vi "LWXPS_SetZone.vi"(5 "LabVIEW error IN":errorcluster, 6 "XPS Reference IN":refnum<k24>, 7 "Hysteresis":dbl, 8 "Radius":dbl, 9 "Y center":dbl, 10 "X center":dbl) -> (0 "LabVIEW error OUT":errorcluster, 1 "XPS Error String":string, 2 "Returned error code":i32, 3 "XPS Reference OUT":refnum<k24>)   [LabVIEW 2014]
uses:
  D:/XPSQ8_LabView_Library/Development/Source/Dll/Newport.XPS.CommandInterface.dll
  Dll/Newport.XPS.CommandInterface.dll
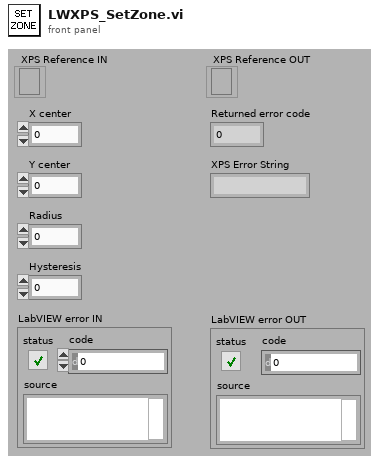
[diagram p1: front panel]
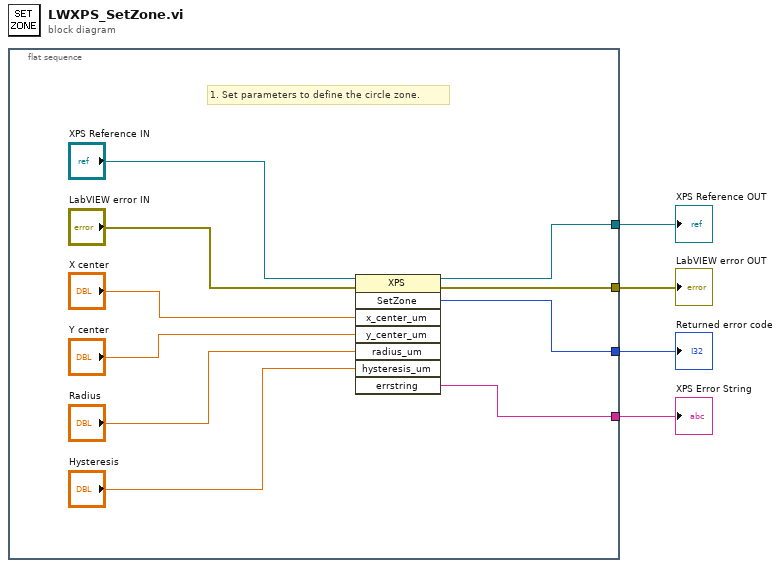
[diagram p0: block diagram]
diagram:
  n1 = flat-sequence {
    tunnel: [w11] -> w4
    tunnel: [w10] -> w3
    tunnel: [w12] -> w2
    tunnel: [w7] -> w1
    frame #0 {
      # "1. Set parameters to define the circle zone."
      n2 = invoke class="XPS" method="SetZone"(reference="XPS Reference IN", error in="LabVIEW error IN", "x_center_um"="X center", "y_center_um"="Y center", "radius_um"="Radius", "hysteresis_um"="Hysteresis") -> (reference out=w11:refnum<k24>, error out=w10:errorcluster, "SetZone"=w12:i32, "errstring"=w7:string)  [unwired: 2 in, 4 out]
    }
  }
  "XPS Error String" <- w1
  "XPS Reference OUT" <- w4
  "LabVIEW error OUT" <- w3
  "Returned error code" <- w2
